vi "mapan.vi"(0 "lwf":dbl, 5 "rwf":dbl, 7 "direct":dbl, 9 "xposit":dbl, 11 "yposit":dbl) -> (4 "xposit 2":dbl, 6 "yposit 2":dbl, 8 "direct 2":dbl)   [LabVIEW 2015]
uses:
  <vilib>/imath/engines/lvmath2/RunTimeEngine/BuiltInFunctions/abs/NIMS_abs(signed).vi
  <instcachedir>/0/NIMS_abs(signed)_C4FCB8E6058B49B797C7C8D53CA5F6EC.lvgen/NIMS_abs(signed)_C4FCB8E6058B49B797C7C8D53CA5F6EC_000.vi
  <vilib>/imath/engines/lvmath2/RunTimeEngine/NodeEndStatement/NIMS_NodeEndStatement_Output.vi
  <instcachedir>/0/NIMS_NodeEndStatement_Output_53EC0D466D134D7ABD903AC30B43404B.lvgen/NIMS_NodeEndStatement_Output_53EC0D466D134D7ABD903AC30B43404B_001.vi
  <vilib>/imath/engines/lvmath2/RunTimeEngine/ErrorHandling/NIMS_Finalize Error.vi
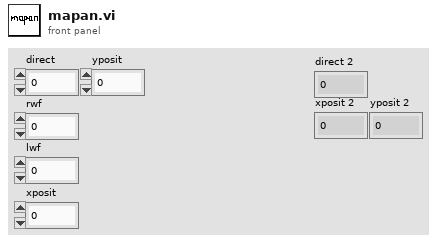
[diagram p1: front panel]
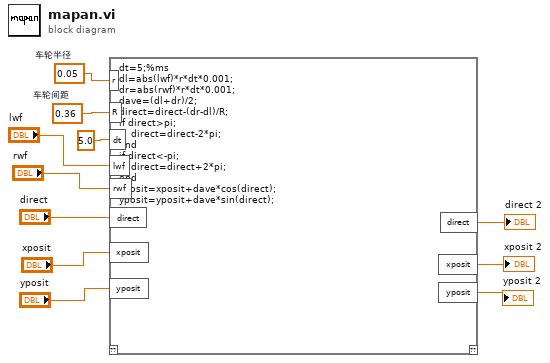
[diagram p0: block diagram]
diagram:
  w6 = 0.05  # 车轮半径
  w7 = 0.36  # 车轮间距
  n1 = mathscript code="dt=5;%ms\ndl=abs(lwf)*r*dt*0.001;\ndr=abs(rwf)*r*dt*0.001;\ndave=(dl+dr)/2;\ndirect=direct-(dr-dl)/R;\nif direct>pi;\n    direct=direct-2*pi;\nend\nif direct<-pi;\n    direct=direct+2*pi;\nend\nxposit=xposit+dave*cos(direct);\nyposit=yposit+dave*sin(direct);"("r"=w6, "R"=w7, "dt"=5.0, "lwf"="lwf", "rwf"="rwf", "direct"="direct", "xposit"="xposit", "yposit"="yposit") -> ("direct"=→"direct 2":dbl, "xposit"=→"xposit 2":dbl, "yposit"=→"yposit 2":dbl)  [unwired: 1 in, 1 out]
